vi "rs3 create context2.vi"(8 "error in (no error)":errorcluster, 11 "version":i32=20000) -> (0 "error out":errorcluster, 3 "context":u32)   [LabVIEW 2017, in "libRealSense3.lvlib"]
doc: "This has to be the first call to initialize libRealSense. \nThe input is the Version Check for the libRealSense, and the output is the Context that needs to be passed to Device Count and Get Device, etc."
uses:
  <vilib>/addons/RealSense/libRealSense3.lvlib
  <vilib>/addons/RealSense/realsense-d.dll
panel:
  # "RS3 Create Context2"
  # "(C) Intel Corp.,  AGJ"
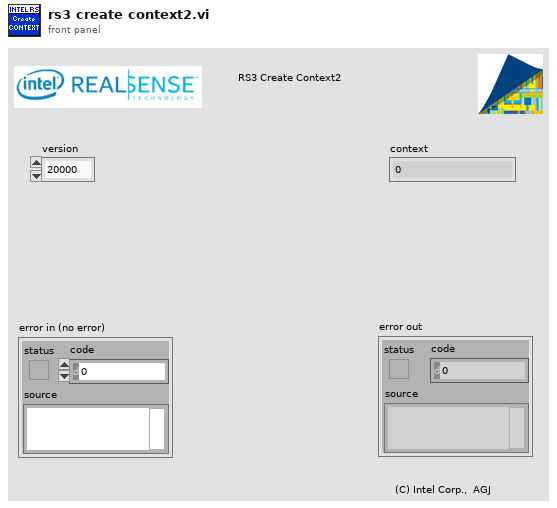
[diagram p1: front panel]
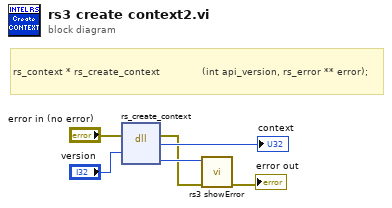
[diagram p0: block diagram]
diagram:
  # "rs_context * rs_create_context              (int api_version, rs_error ** error);"
  n1 = dll-call lib="C:/Program Files (x86)/National Instruments/LabVIEW 2017/vi.lib/addons/RealSense/realsense-d.dll" fn="rs_create_context"(error in="error in (no error)", "api_version"="version") -> (error out=w1:errorcluster, "context"=→"context":u64, "error"=w2:u64)  [unwired: 4 in, 1 out]
  n2 = call <vilib>:"rs3 showError.vi"("error in (no error)"=w1, "error"=w2) -> ("error out"=→"error out":errorcluster)  [unwired: 5 in, 4 out]
